vi "Add Proto Search Path.vi"(8 "error in (no error)":errorcluster, 10 "Search Path":path, 11 "protoFile ref in":u64) -> (0 "error out":errorcluster, 3 "protoFile ref out":u64)   [LabVIEW 2019, in "gRPC Template Creation Utility.lvlib"]
uses:
  gRPC Template Creation Utility.lvlib
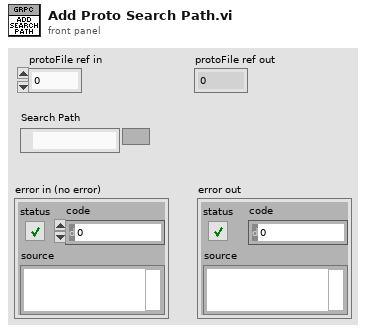
[diagram p1: front panel]
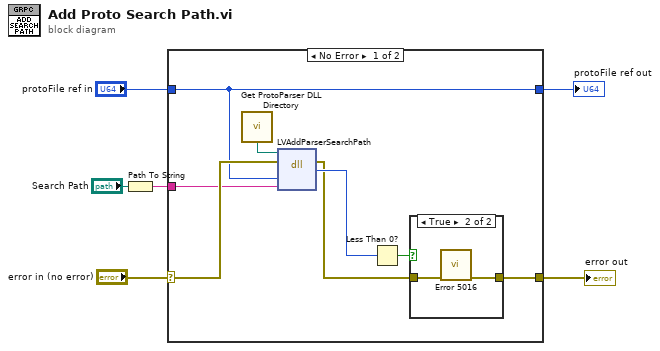
[diagram p0: block diagram]
diagram:
  n1 = Path To String(path="Search Path") -> (string=w1:string)
  n2 = case shown="No Error" "error in (no error)" {
    selector: "error in (no error)" -> [w13 w19]
    tunnel: "protoFile ref in" -> [w12 w18]
    tunnel: [w8 w19] -> w4
    tunnel: [w12 w18] -> w5
    tunnel: w1 -> [w7 _]
    frame No Error {
      n3 = call "Get ProtoParser DLL Directory.vi"() -> ("Proto Parser Directory"=w14:path)
      n4 = dll-call lib="?" fn="LVAddParserSearchPath"(path in=w14, error in=w13, "protoRef"=w12, "searchPath"=w7) -> (error out=w9:errorcluster, "return type"=w11:i32)  [unwired: 3 in, 1 out]
      n5 = Less Than 0?(x=w11) -> (x < 0?=w10:bool)
      n6 = case shown="True" w10 {
        tunnel: w9 -> [w15 w17]
        tunnel: [w15 w16] -> w8
        frame False {
        }
        frame True {
          n7 = call "Error 5016.vi"("error in (no error)"=w17) -> ("error out"=w16:errorcluster)  [unwired: 10 in]
        }
      }
    }
    frame Error {
    }
  }
  "protoFile ref out" <- w5
  "error out" <- w4
